vi "Maquina Expendedora.vi"() -> ()   [LabVIEW 2020]
doc: "Esta es una maquina expendedora de Cheetos, Nitos, Coca cola, usted introduce el dinero, decide cuantos productos se desean, devuelve el dinero a pagar, te dice si esta funcionando o no"
panel:
  out "Nitos?":bool
  out "Coca?":bool
  out "Cheetos?":bool
  out "Devuelve de a 50 Peso":i16 min=0
  out "Devuelve de a 20 Peso":i16 min=0
  out "Devuelve de a 10 Peso":i16 min=0
  out "Devuelve de a 5 Peso":i16 min=0
  out "Devuelve de a 2 Peso":i16 min=0
  out "Devuelve de a Peso":i16 min=0
  out "Cambio:":dbl
  out "Dinero a pagar:":dbl
  in  "Cantidad Nitos":i8 min=0
  in  "Cantidad Coca":i8 min=0
  out "Funcionando?":bool
  out "Dinero ingresado:":dbl
  in  "Billetes de 50 Pesos":i16 min=0
  in  "Billetes de 20 Pesos":i16 min=0
  in  "Monedas de a 10 Pesos":i16 min=0
  in  "Monedas de a 5 Pesos":i16 min=0
  in  "Monedas de a 2 Pesos":i16 min=0
  in  "Monedas de a Peso":i16 min=0
  in  "Cantidad Cheetos":i8 min=0
  out "Estado: .":string
  # "Monedas y billetes que la\nmaquina acepta."
  # "Esto es donde cada uno elige sus productos"
  # "Cheetos Flamin' Hot"
  # "Coca - Cola"
  # "Precio: 15$"
  # "Precio: 12$"
  # "2 Nitos Bimbo"
  # "Precio: 22$"
  # "Aquí devuelve el cambio"
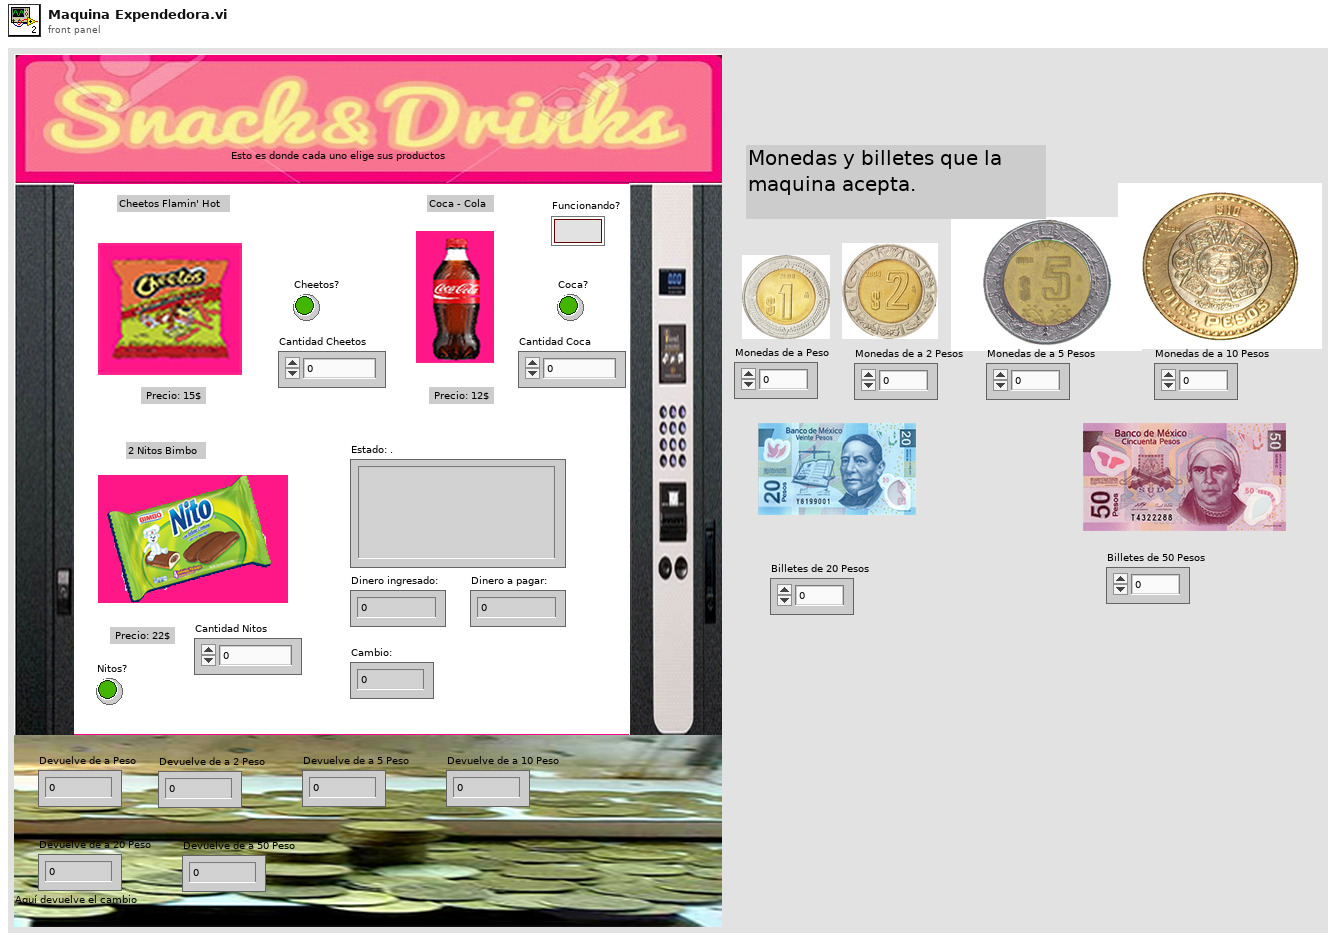
[diagram p1: front panel]
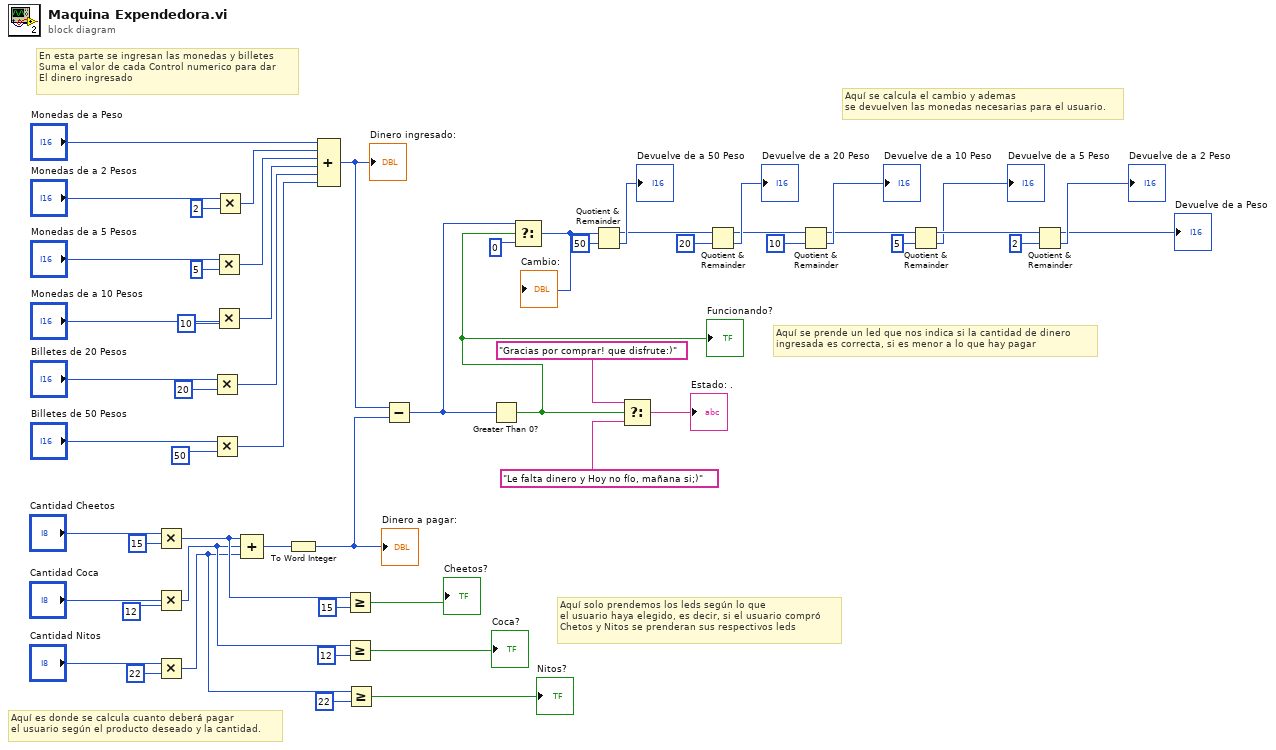
[diagram p0: block diagram]
diagram:
  # "Aquí solo prendemos los leds según lo que\nel usuario haya elegido, es decir, si el usuario compró\nChetos y Nitos se prenderan sus respectivos leds"
  # "Aquí se prende un led que nos indica si la cantidad de dinero\ningresada es correcta, si es menor a lo que hay pagar"
  # "Aquí se calcula el cambio y ademas\nse devuelven las monedas necesarias para el usuario."
  # "Aquí es donde se calcula cuanto deberá pagar\nel usuario según el producto deseado y la cantidad."
  # "En esta parte se ingresan las monedas y billetes\nSuma el valor de cada Control numerico para dar\nEl dinero ingresado"
  n1 = Multiply(x="Cantidad Cheetos", y=i8 15) -> (x*y=w9:i8)
  n2 = Multiply(x="Cantidad Coca", y=i8 12) -> (x*y=w7:i8)
  n3 = Multiply(x="Cantidad Nitos", y=i8 22) -> (x*y=w5:i8)
  n4 = Multiply(x="Billetes de 20 Pesos", y=i16 20) -> (x*y=w42:i16)
  n5 = Multiply(x="Billetes de 50 Pesos", y=i16 50) -> (x*y=w41:i16)
  n6 = Multiply(x="Monedas de a 5 Pesos", y=i16 5) -> (x*y=w44:i16)
  n7 = Multiply(x="Monedas de a 10 Pesos", y=i16 10) -> (x*y=w43:i16)
  n8 = Multiply(x="Monedas de a 2 Pesos", y=i16 2) -> (x*y=w45:i16)
  n9 = Compound Arithmetic op=ADD(w9, w7, w5) -> (w10:i8)
  n10 = To Word Integer(number=w10) -> (16bit integer=w11:i16)
  "Dinero a pagar:" <- w11
  n11 = Compound Arithmetic op=ADD("Monedas de a Peso", w45, w44, w43, w42, w41) -> (w34:i16)
  "Dinero ingresado:" <- w34
  n12 = Greater Or Equal?(x=w9, y=i8 15) -> (x >= y?=→"Cheetos?":bool)
  n13 = Greater Or Equal?(x=w7, y=i8 12) -> (x >= y?=→"Coca?":bool)
  n14 = Greater Or Equal?(x=w5, y=i8 22) -> (x >= y?=→"Nitos?":bool)
  n15 = Subtract(x=w34, y=w11) -> (x-y=w29:i16)
  n16 = Greater Than 0?(x=w29) -> (x > 0?=w30:bool)
  "Funcionando?" <- w30
  n17 = Select(t=w29, s=w30, f=i16 0) -> (s? t:f=w27:i16)
  "Cambio:" <- w27
  n18 = Quotient & Remainder(x=w27, y=i16 50) -> (x-y*floor(x/y)=w20:i16, floor(x/y)=→"Devuelve de a 50 Peso":i16)
  n19 = Select(t="Gracias por comprar! que disfrute:)", s=w30, f="Le falta dinero y Hoy no fío, mañana si;)") -> (s? t:f=→"Estado: .":string)
  n20 = Quotient & Remainder(x=w20, y=i16 20) -> (x-y*floor(x/y)=w18:i16, floor(x/y)=→"Devuelve de a 20 Peso":i16)
  n21 = Quotient & Remainder(x=w18, y=i16 10) -> (x-y*floor(x/y)=w16:i16, floor(x/y)=→"Devuelve de a 10 Peso":i16)
  n22 = Quotient & Remainder(x=w16, y=i16 5) -> (x-y*floor(x/y)=w15:i16, floor(x/y)=→"Devuelve de a 5 Peso":i16)
  n23 = Quotient & Remainder(x=w15, y=i16 2) -> (x-y*floor(x/y)=→"Devuelve de a Peso":i16, floor(x/y)=→"Devuelve de a 2 Peso":i16)
